vi "Main (1).vi"() -> ()   [LabVIEW 2015]
uses:
  <vilib>/express/express analysis/Spectral/XNode/ExpressSpectralMeasurementsBlockNode.xnode
  <vilib>/express/express analysis/Spectral/Block/exnSpectralBlock spectral measurements power poly.vi
  <vilib>/measure/NI_MABase.lvlib
  <vilib>/express/express analysis/Spectral/Block/exnSpectralBlock spectral measurements power DDT.vi
panel:
  in  "Blue Offset":dbl
  in  "Green Offset":dbl
  in  "Red Offset":dbl
  in  "?":bool
  in  "?":bool
  in  "?":bool
  out "Green RGB":i16
  out "Blue RGB":i16
  out "Red RGB":i16
  out "Blue\nPower":dbl
  in  "Blue\nFrequency":dbl
  out "Green\nPower":dbl
  in  "Green\nFrequency":dbl
  out "Red\nPower":dbl
  in  "Red\nFrequency":dbl
  out "Color":u32(colorbox)
  out "Timestream":dynamicdata(graph)
  out "Power Spectrum":dynamicdata(graph)
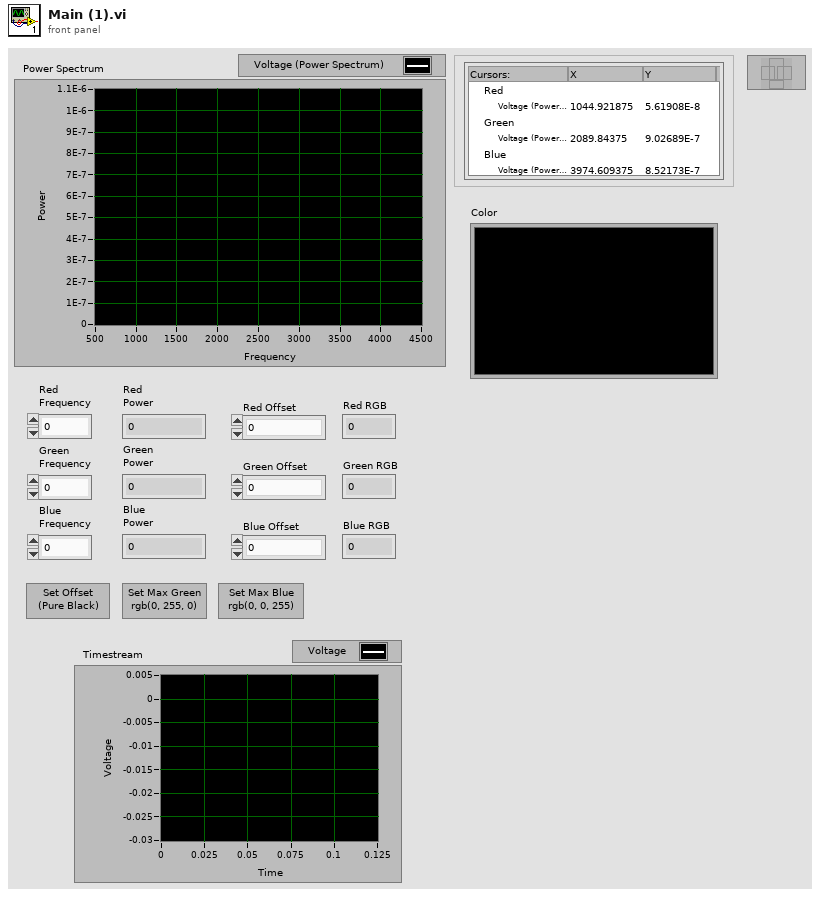
[diagram p1: front panel]
types:
  T1 = cluster{"averaging mode":u16, "weighting mode":u16, "number of averages":u32}
  T2 = cluster{"dB On (F)":bool, "unwrap phase (F)":bool, "convert to degree (F)":bool}
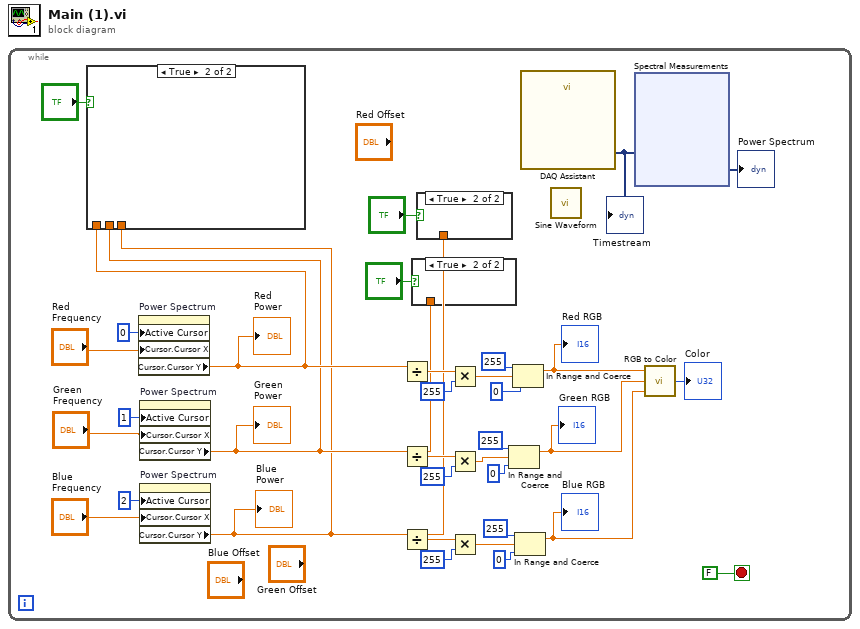
[diagram p0: block diagram]
diagram:
  n1 = while {
    stop <- FALSE stop-if-true
    n2 = property on="Power Spectrum" class="WFGraph (strict)"("Active Cursor"=u32 0, "Cursor.Cursor X"="Red\nFrequency") -> ("Cursor.Cursor Y"=w17:dbl)  [unwired: 2 in, 2 out]
    "Red\nPower" <- w17
    n3 = property on="Power Spectrum" class="WFGraph (strict)"("Active Cursor"=u32 1, "Cursor.Cursor X"="Green\nFrequency") -> ("Cursor.Cursor Y"=w2:dbl)  [unwired: 2 in, 2 out]
    "Green\nPower" <- w2
    n4 = property on="Power Spectrum" class="WFGraph (strict)"("Active Cursor"=u32 2, "Cursor.Cursor X"="Blue\nFrequency") -> ("Cursor.Cursor Y"=w1:dbl)  [unwired: 2 in, 2 out]
    "Blue\nPower" <- w1
    n5 = case shown="True" "?" {
      tunnel: w17 -> [_ _]
      tunnel: w2 -> [_ _]
      tunnel: w1 -> [_ _]
      frame False {
      }
      frame True {
      }
    }
    n6 = Divide(x=w17) -> (x/y=w33:dbl)  [unwired: 1 in]
    n7 = Divide(x=w2) -> (x/y=w30:dbl)  [unwired: 1 in]
    n8 = Divide(x=w1) -> (x/y=w28:dbl)  [unwired: 1 in]
    n9 = case shown="True" "?" {
      tunnel: w2 -> [_ _]
      frame False {
      }
      frame True {
      }
    }
    n10 = case shown="True" "?" {
      tunnel: w1 -> [_ _]
      frame False {
      }
      frame True {
      }
    }
    n11 = Multiply(x=w33, y=255) -> (x*y=w8:dbl)
    n12 = Multiply(x=w30, y=255) -> (x*y=w6:dbl)
    n13 = Multiply(x=w28, y=255) -> (x*y=w4:dbl)
    n14 = In Range and Coerce(upper limit=i16 255, x=w6, lower limit=i16 0) -> (coerced(x)=w5:dbl)  [unwired: 1 out]
    "Green RGB" <- w5
    n15 = In Range and Coerce(upper limit=i16 255, x=w8, lower limit=i16 0) -> (coerced(x)=w7:dbl)  [unwired: 1 out]
    "Red RGB" <- w7
    n16 = In Range and Coerce(upper limit=i16 255, x=w4, lower limit=i16 0) -> (coerced(x)=w3:dbl)  [unwired: 1 out]
    "Blue RGB" <- w3
    n17 = call "DAQ Assistant"() -> ("data"=w26:dynamicdata)  [unwired: 17 in, 2 out]
    "Timestream" <- w26
    n18 = call <vilib>:"Sine Waveform.vi"() -> ()  [unwired: 10 in, 2 out]
    n19 = xnode "Spectral Measurements"("Signals"=w26) -> ("Power Spectrum"=→"Power Spectrum":dynamicdata)  [unwired: 1 in, 1 out]
    n20 = call <vilib>:"RGB to Color.vi"("B"=w3, "G"=w5, "R"=w7) -> ("Color"=→"Color":u32)
  }
